vi "solar tracking.vi"() -> ()   [LabVIEW 2020]
uses:
  <vilib>/LabVIEW Interface for Arduino/Type Defs/Connection Type.ctl
  <vilib>/LabVIEW Interface for Arduino/Type Defs/Board Type.ctl
  <vilib>/LabVIEW Interface for Arduino/LabVIEW Interface for Arduino.lvlib
panel:
  in  "bottom motor":dbl(knob) scale=0.0..180.0
  out "dirction bottom":dbl(knob) scale=0.0..360.0
  out "voltage 2":dbl
  in  "?":dbl(knob) scale=0.0..180.0
  out "dirction top":dbl(knob) scale=-45.0..45.0
  out "o/p solar panel":dbl(graph)
  in  "type control":bool
  in  "VISA resource":refnum<visa-resource-name>
  out "LDR 4":dbl
  out "LDR 3":dbl
  out "error out":errorcluster
  in  "stop":bool
  out "LDR 1":dbl
  out "LDR 2":dbl
  # "A"
  # "M"
  # "top motor"
  # "bottom motor"
  # "top motor"
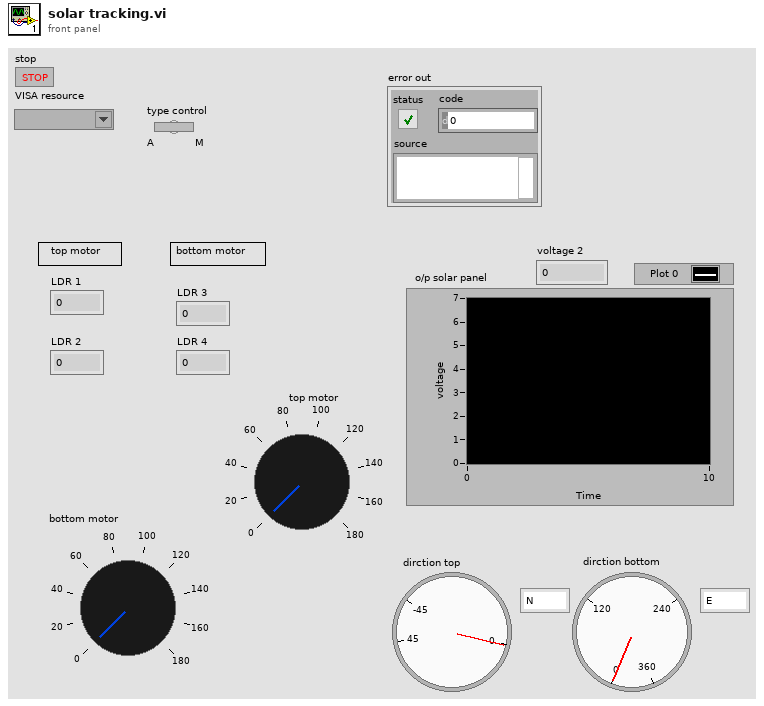
[diagram p1: front panel]
types:
  T1 = typedef "LabVIEW Interface for Arduino.lvlib/Board Type.ctl" = enum16{"Uno", "Dimuelanove w/Atmega 328", "Mega 2560"}
  T2 = typedef "LabVIEW Interface for Arduino.lvlib/Connection Type.ctl" = enum8{"USB / Serial", "XBEE", "BlueSmirf (Bluetooth)"}
  T3 = typedef "LabVIEW Interface for Arduino.lvlib/Arduino Resource.ctl" = cluster{"VISA resource":refnum<visa-resource-name>, "Board Type":T1, "Connection Type":enum8{"USB / Serial"}, "Bytes Per Packet (15)":u8}
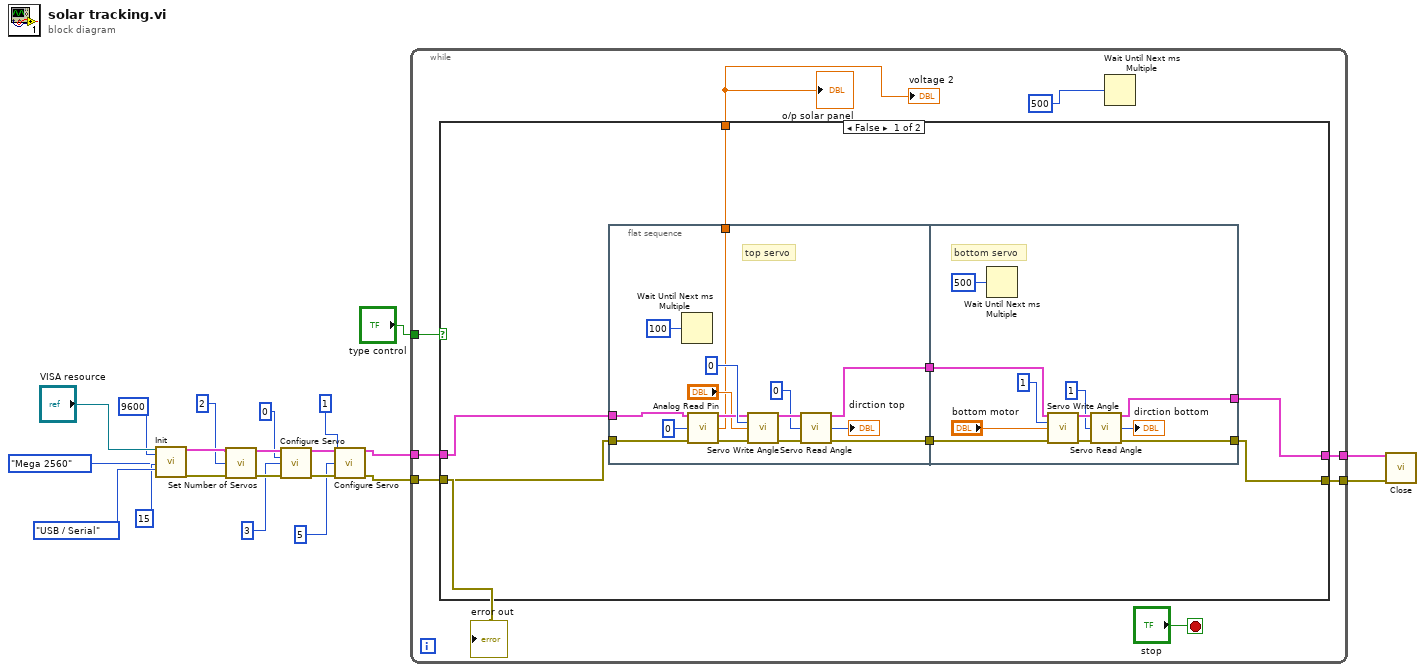
[diagram p0: block diagram]
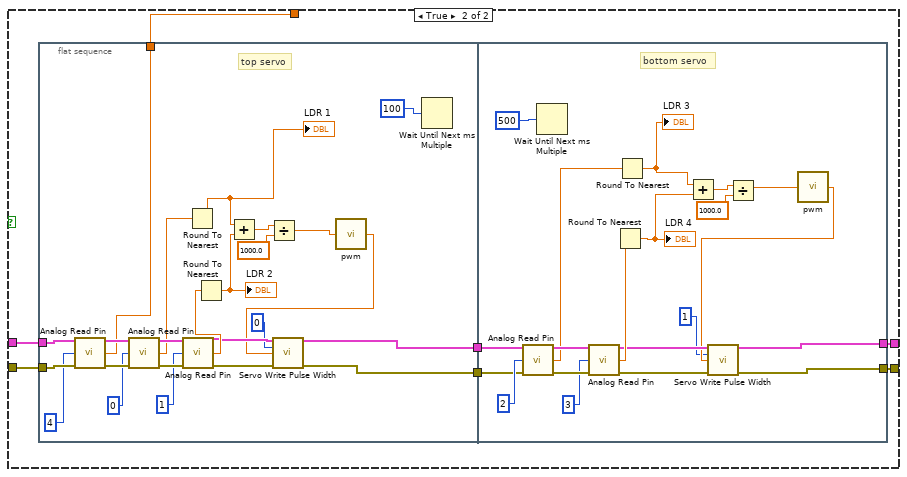
[diagram p2: hidden frame]
diagram:
  n1 = call <vilib>:"Init.vi"("VISA resource"="VISA resource", "Baud Rate (115200)"=u32 9600, "Board Type (Uno)"=Board_Type."Mega 2560", "Bytes Per Packet (15)"=u32 15, "Connection Type (USB/Serial)"=Connection_Type."USB / Serial") -> ("Arduino Resource"=w21:T3, "error out"=w16:errorcluster)  [unwired: 13 in]
  n2 = call <vilib>:"Set Number of Servos.vi"("Arduino Resource"=w21, "Number Of Servos (1)"=u8 2, "error in"=w16) -> ("Arduino Resource"=w20:T3, "error out"=w19:errorcluster)  [unwired: 11 in]
  n3 = call <vilib>:"Configure Servo.vi"("Arduino Resource"=w20, "Servo Number (0)"=u8 0, "DIO Pin (2)"=u8 3, "error in"=w19) -> ("Arduino Resource"=w18:T3, "error out"=w17:errorcluster)  [unwired: 10 in]
  n4 = call <vilib>:"Configure Servo.vi"("Arduino Resource"=w18, "Servo Number (0)"=u8 1, "DIO Pin (2)"=u8 5, "error in"=w17) -> ("Arduino Resource"=w14:T3, "error out"=w15:errorcluster)  [unwired: 10 in]
  n5 = while {
    tunnel: w14 -> [w29]
    tunnel: w15 -> [w27]
    tunnel: [w26] -> w7
    tunnel: [w25] -> w6
    tunnel: "type control" -> [w24]
    stop <- "stop" stop-if-true
    n6 = case shown="False" w24 {
      tunnel: w29 -> [w34 w67]
      tunnel: w27 -> [w33 w66]
      tunnel: [w32 w65] -> w26
      tunnel: [w31 w64] -> w25
      tunnel: [w30 w63] -> w22
      frame False {
        n7 = flat-sequence {
          tunnel: w34 -> [w50]
          tunnel: w33 -> [w49]
          tunnel: [w45] -> w36
          tunnel: [w44] -> w35
          tunnel: [w37] -> w30
          tunnel: w36 -> [w57]
          tunnel: w35 -> [w56]
          tunnel: [w59] -> w32
          tunnel: [w58] -> w31
          frame #0 {
            # "top servo"
            n8 = Wait Until Next ms Multiple(millisecond multiple=u32 100) -> ()  [unwired: 1 out]
            n9 = call <vilib>:"Analog Read Pin.vi"("Arduino Resource"=w50, "Analog Input Pin (0)"=u8 0, "error in"=w49) -> ("Arduino Resource"=w41:T3, "Voltage"=w37:dbl, "error out"=w40:errorcluster)  [unwired: 10 in]
            n10 = call <vilib>:"Servo Write Angle.vi"("Arduino Resource"=w41, "Servo Number"=u8 0, "Angle (Degrees)"="?", "error in"=w40) -> ("Arduino Resource"=w47:T3, "error out"=w46:errorcluster)  [unwired: 10 in]
            n11 = call <vilib>:"Servo Read Angle.vi"("Arduino Resource"=w47, "Servo Number"=u8 0, "error in"=w46) -> ("Arduino Resource"=w45:T3, "Angle (Degrees)"=→"dirction top":u8, "error out"=w44:errorcluster)  [unwired: 10 in]
          }
          frame #1 {
            # "bottom servo"
            n12 = Wait Until Next ms Multiple(millisecond multiple=u32 500) -> ()  [unwired: 1 out]
            n13 = call <vilib>:"Servo Write Angle.vi"("Arduino Resource"=w57, "Servo Number"=u8 1, "Angle (Degrees)"="bottom motor", "error in"=w56) -> ("Arduino Resource"=w61:T3, "error out"=w60:errorcluster)  [unwired: 10 in]
            n14 = call <vilib>:"Servo Read Angle.vi"("Arduino Resource"=w61, "Servo Number"=u8 1, "error in"=w60) -> ("Arduino Resource"=w59:T3, "Angle (Degrees)"=→"dirction bottom":u8, "error out"=w58:errorcluster)  [unwired: 10 in]
          }
        }
      }
      frame True {
        n15 = flat-sequence {
          tunnel: w67 -> [w87]
          tunnel: w66 -> [w86]
          tunnel: [w74] -> w69
          tunnel: [w73] -> w68
          tunnel: [w70] -> w63
          tunnel: w69 -> [w106]
          tunnel: w68 -> [w105]
          tunnel: [w98] -> w65
          tunnel: [w97] -> w64
          frame #0 {
            # "top servo"
            n16 = call <vilib>:"Analog Read Pin.vi"("Arduino Resource"=w87, "Analog Input Pin (0)"=u8 4, "error in"=w86) -> ("Arduino Resource"=w88:T3, "Voltage"=w70:dbl, "error out"=w89:errorcluster)  [unwired: 10 in]
            n17 = call <vilib>:"Analog Read Pin.vi"("Arduino Resource"=w88, "Analog Input Pin (0)"=u8 0, "error in"=w89) -> ("Arduino Resource"=w93:T3, "Voltage"=w79:dbl, "error out"=w92:errorcluster)  [unwired: 10 in]
            n18 = call <vilib>:"Analog Read Pin.vi"("Arduino Resource"=w93, "Analog Input Pin (0)"=u8 1, "error in"=w92) -> ("Arduino Resource"=w82:T3, "Voltage"=w90:dbl, "error out"=w81:errorcluster)  [unwired: 10 in]
            n19 = Round To Nearest(number=w79) -> (nearest integer value=w78:dbl)
            "LDR 1" <- w78
            n20 = Round To Nearest(number=w90) -> (nearest integer value=w77:dbl)
            "LDR 2" <- w77
            n21 = Add(x=w78, y=w77) -> (x+y=w76:dbl)
            n22 = Divide(x=w76, y=1000.0) -> (x/y=w72:dbl)
            n23 = call "pwm.vi"("Analog Signal"=w72) -> ("Numeric"=w71:dbl)
            n24 = call <vilib>:"Servo Write Pulse Width.vi"("Arduino Resource"=w82, "Servo Number"=u8 0, "Pulse Width in uS"=w71, "error in"=w81) -> ("Arduino Resource"=w74:T3, "error out"=w73:errorcluster)  [unwired: 10 in]
            n25 = Wait Until Next ms Multiple(millisecond multiple=u32 100) -> ()  [unwired: 1 out]
          }
          frame #1 {
            # "bottom servo"
            n26 = call <vilib>:"Analog Read Pin.vi"("Arduino Resource"=w106, "Analog Input Pin (0)"=u8 2, "error in"=w105) -> ("Arduino Resource"=w111:T3, "Voltage"=w110:dbl, "error out"=w112:errorcluster)  [unwired: 10 in]
            n27 = Wait Until Next ms Multiple(millisecond multiple=u32 500) -> ()  [unwired: 1 out]
            n28 = call <vilib>:"Analog Read Pin.vi"("Arduino Resource"=w111, "Analog Input Pin (0)"=u8 3, "error in"=w112) -> ("Arduino Resource"=w104:T3, "Voltage"=w109:dbl, "error out"=w103:errorcluster)  [unwired: 10 in]
            n29 = Round To Nearest(number=w109) -> (nearest integer value=w100:dbl)
            "LDR 4" <- w100
            n30 = Round To Nearest(number=w110) -> (nearest integer value=w99:dbl)
            "LDR 3" <- w99
            n31 = Add(x=w99, y=w100) -> (x+y=w102:dbl)
            n32 = Divide(x=w102, y=1000.0) -> (x/y=w96:dbl)
            n33 = call "pwm.vi"("Analog Signal"=w96) -> ("Numeric"=w95:dbl)
            n34 = call <vilib>:"Servo Write Pulse Width.vi"("Arduino Resource"=w104, "Servo Number"=u8 1, "Pulse Width in uS"=w95, "error in"=w103) -> ("Arduino Resource"=w98:T3, "error out"=w97:errorcluster)  [unwired: 10 in]
          }
        }
      }
    }
    "o/p solar panel" <- w22
    "voltage 2" <- w22
    n35 = Wait Until Next ms Multiple(millisecond multiple=u32 500) -> ()  [unwired: 1 out]
    "error out" <- w27
  }
  n36 = call <vilib>:"Close.vi"("Arduino Resource"=w7, "error in"=w6) -> ()  [unwired: 13 in, 1 out]
